vi "Get USB COMport_device_hub_and_port_numbers .vi"() -> ()   [LabVIEW 2013]
uses:
  <vilib>/Utility/file.llb/Read From Spreadsheet File (string).vi
panel:
  in  "PID":string
  in  "VID":string
  in  "Filter by VID_PID?":bool=TRUE
  out "error out":errorcluster
  out "standard output":string
  in  "error in (no error)":errorcluster
  out "Matching COMPORT Devices":i32
  out "Array":string[][](array[string])
  out "all rows":string[][](array[string])
  in  "file path (dialog if empty)":path=path "L:/junk2.csv"
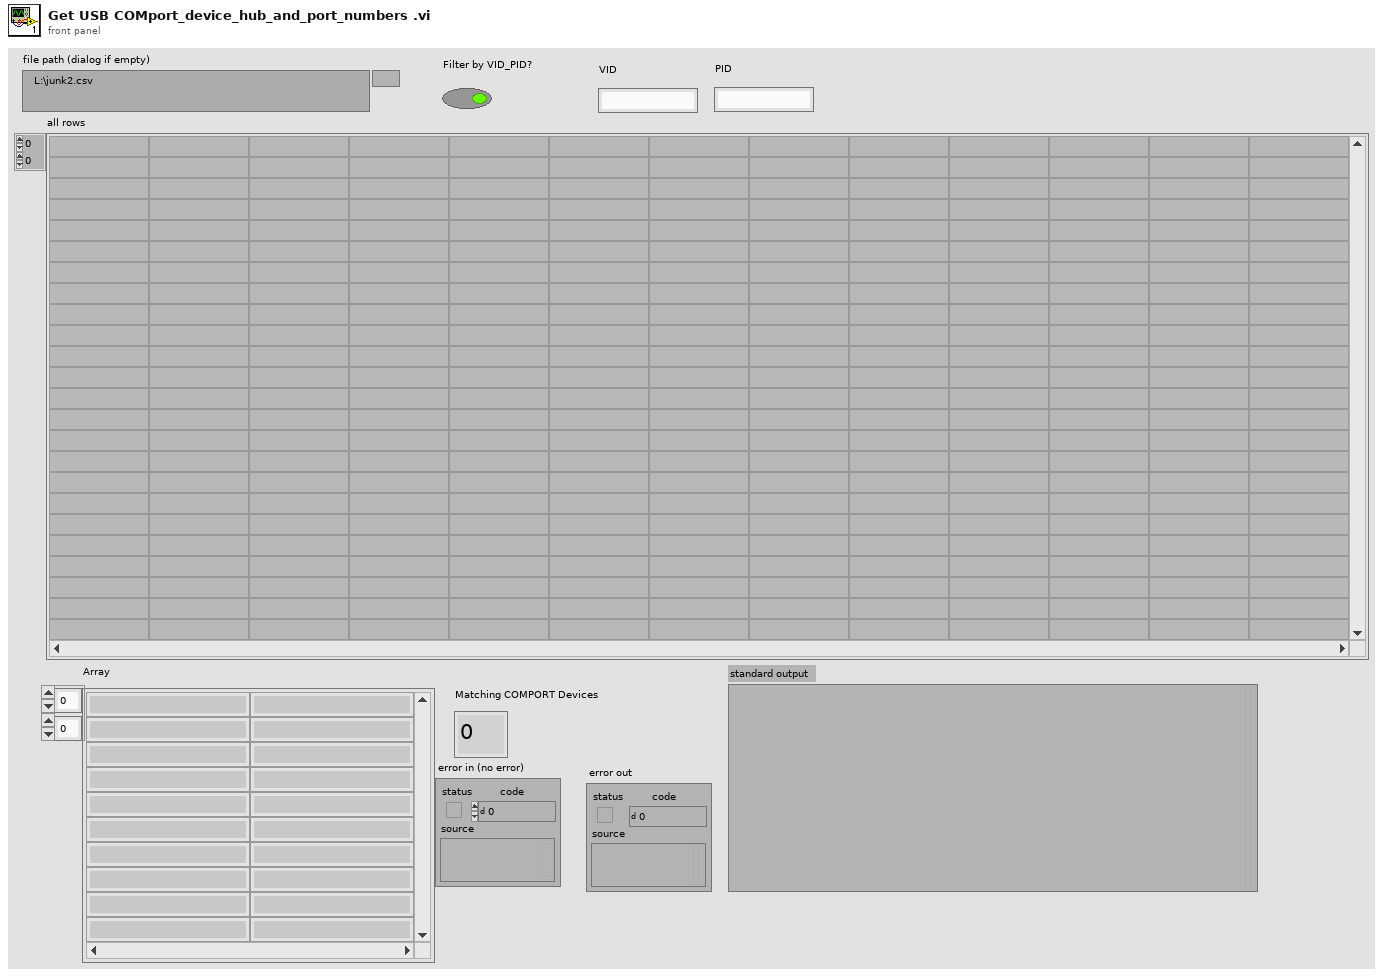
[diagram p1: front panel]
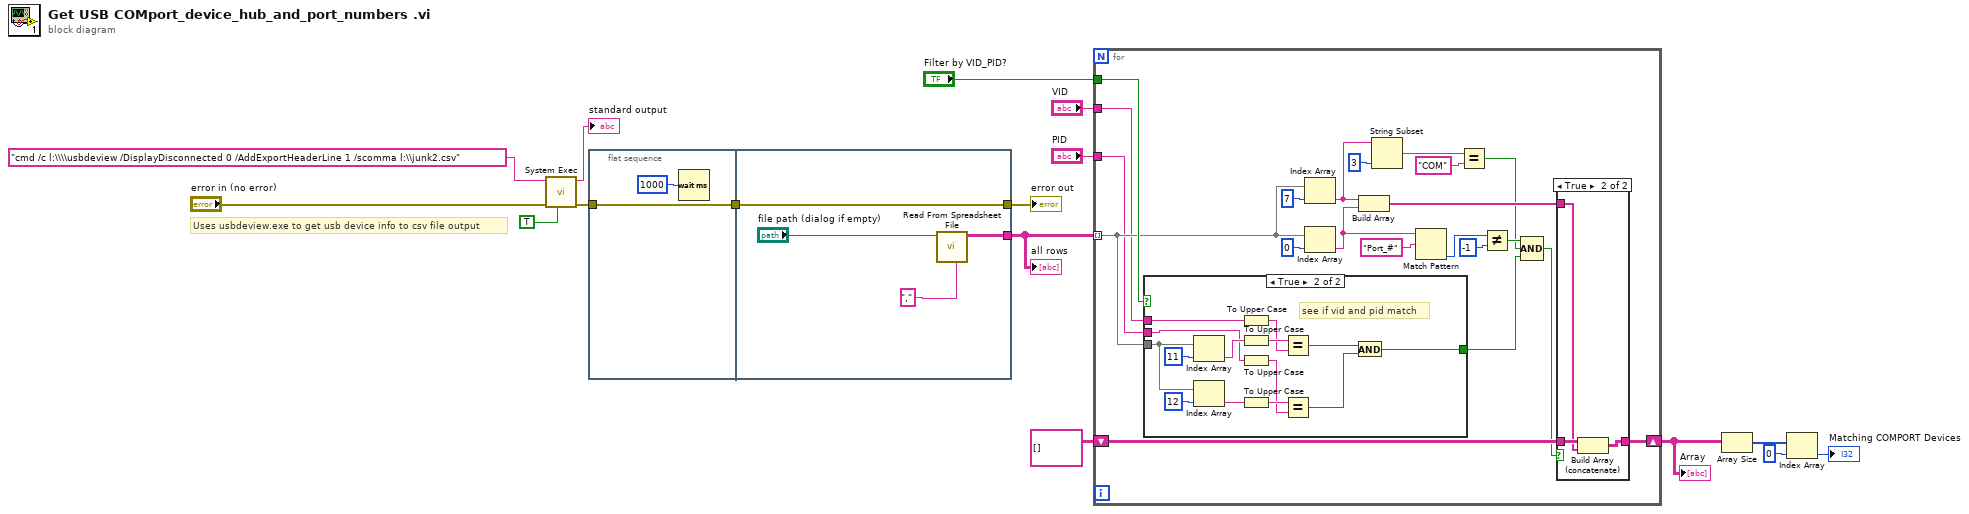
[diagram p0: block diagram]
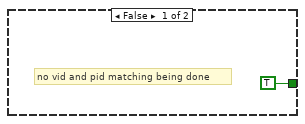
[diagram p2: hidden frame]
diagram:
  # "Uses usbdeview.exe to get usb device info to csv file output"
  n1 = call <vilib>:"System Exec.vi"("run minimized? (F)"=TRUE, "error in (no error)"="error in (no error)", "command line"="cmd /c l:\\\\usbdeview /DisplayDisconnected 0 /AddExportHeaderLine 1 /scomma l:\\junk2.csv") -> ("error out"=w5:errorcluster, "standard output"=→"standard output":string)  [unwired: 5 in, 2 out]
  n2 = flat-sequence {
    tunnel: w5 -> [w18]
    tunnel: [w18] -> w4
    tunnel: [w20] -> w16
    tunnel: [w19] -> w6
    tunnel: w4 -> [w19]
    frame #0 {
      n3 = Wait (ms)(milliseconds to wait=u32 1000) -> ()  [unwired: 1 out]
    }
    frame #1 {
      n4 = call-poly <vilib>:"Read From Spreadsheet File.vi"("delimiter (\\t)"="," ("delimiter (\\t)"), "file path (dialog if empty)"="file path (dialog if empty)") -> ("all rows"=w20:string[][])  [unwired: 5 in, 4 out]
    }
  }
  n5 = for {
    tunnel: w16 -> [w29] mode=indexing
    shift-right: [w36] -> w14
    shift-left: string[][] [] -> [w39]
    tunnel: "Filter by VID_PID?" -> [w30]
    tunnel: "VID" -> [w28]
    tunnel: "PID" -> [w27]
    n6 = case shown="True" w30 {
      tunnel: w29 -> [_ w58]
      tunnel: w28 -> [_ w53]
      tunnel: w27 -> [_ w52]
      tunnel: [TRUE w45] -> w24
      frame False {
        # "no vid and pid matching being done"
      }
      frame True {
        # "see if vid and pid match"
        n7 = Index Array(array=w58, index=11) -> (element=w55:string)
        n8 = Index Array(array=w58, index=12) -> (element=w54:string)
        n9 = To Upper Case(1:w53) -> (0:w50:string)
        n10 = To Upper Case(1:w55) -> (0:w51:string)
        n11 = To Upper Case(1:w52) -> (0:w48:string)
        n12 = To Upper Case(1:w54) -> (0:w49:string)
        n13 = Equal?(x=w51, y=w50) -> (x = y?=w47:bool)
        n14 = Equal?(x=w49, y=w48) -> (x = y?=w46:bool)
        n15 = And(x=w47, y=w46) -> (x .and. y?=w45:bool)
      }
    }
    n16 = Index Array(array=w29, index=7) -> (element=w32:string)
    n17 = Index Array(array=w29, index=0) -> (element=w31:string)
    n18 = Build Array(w32, w31) -> (w37:string[])
    n19 = String Subset(string=w32, length (rest)=3 ("length (rest)")) -> (substring=w34:string)  [unwired: 1 in]
    n20 = Match Pattern(string=w31, regular expression="Port_#") -> (offset past match=w41:i32)  [unwired: 1 in, 3 out]
    n21 = Equal?(x=w34, y="COM") -> (x = y?=w25:bool)
    n22 = Not Equal?(x=w41, y=-1) -> (x != y?=w26:bool)
    n23 = Compound Arithmetic op=AND(w26, w25, w24) -> (w23:bool)
    n24 = case shown="True" w23 {
      tunnel: w39 -> [w59 w62]
      tunnel: w37 -> [_ w61]
      tunnel: [w59 w60] -> w36
      frame False {
      }
      frame True {
        n25 = Build Array (concatenate)(w62, w61) -> (w60:string[][])
      }
    }
  }
  "Array" <- w14
  n26 = Array Size(array=w14) -> (size(s)=w13:i32[])
  n27 = Index Array(array=w13, index=0) -> (element=→"Matching COMPORT Devices":i32)
  "all rows" <- w16
  "error out" <- w6
